vi "_Axis_Start.vi"(8 "Error In":errorcluster, 11 "轴序号":u16) -> (0 "Error Out":errorcluster)   [LabVIEW 2020, in "MT_API.lvlib"]
doc: "MT_API INT32 __stdcall MT_Set_Axis_Mode_Position_Open(WORD AObj);"
uses:
  MT_API.lvlib
  MT_API_64.dll
panel:
  out "函数返回值":i32
  # "打开当前轴位置模式"
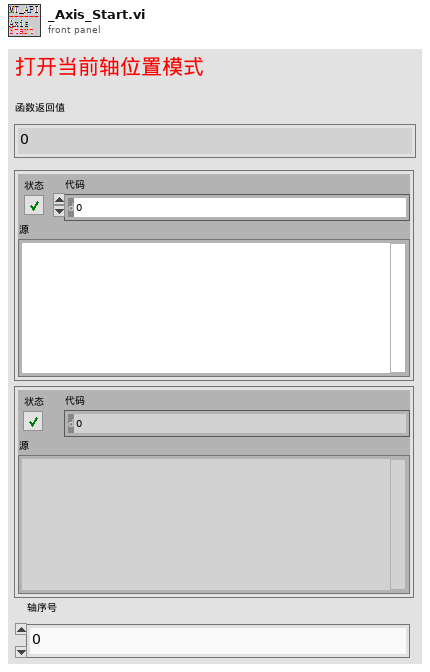
[diagram p1: front panel]
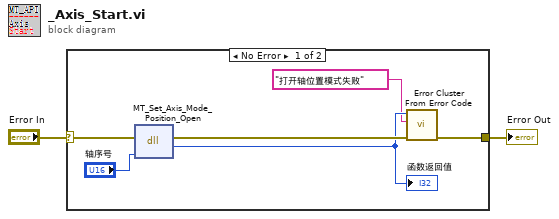
[diagram p0: block diagram]
diagram:
  n1 = case shown="No Error" "Error In" {
    selector: "Error In" -> [w8 w9]
    tunnel: [w4 w9] -> w1
    frame No Error {
      n2 = dll-call lib="D:/Project NJU/lib/MT/MT_API_64.*" fn="MT_Set_Axis_Mode_Position_Open"(error in=w8, "AObj"="轴序号") -> (error out=w6:errorcluster, "return type"=w5:i32)  [unwired: 3 in, 1 out]
      "函数返回值" <- w5
      n3 = call <vilib>:"Error Cluster From Error Code.vi"("error in (no error)"=w6, "error message (\"\")"="打开轴位置模式失败", "error code (0)"=w5) -> ("error out"=w4:errorcluster)  [unwired: 6 in]
    }
    frame Error {
    }
  }
  "Error Out" <- w1
